vi "LC-MISDK_UserCalibration_MakeListData_XYZ.vi"(6 "Before_2":dbl, 7 "Before_3":dbl, 9 "before_1":dbl, 10 "タイムスタンプ":timestamp, 11 "Value":T1(ring)) -> (2 "リファレンス出力":refnum<k24>, 3 ".NET refnum出力":refnum<k24>)   [LabVIEW 2015]
uses:
  C:/Users/e09031/Documents/GMA/LC-160/Labview/Sample_LC-MISDK/LC-MISDK.dll
  LC-MISDK.dll
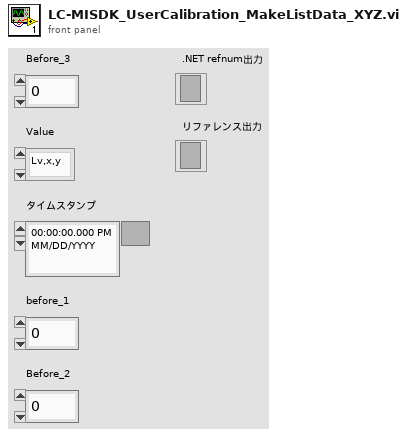
[diagram p1: front panel]
types:
  T1 = enum16{"Lv,x,y", "Lv,u',v'", "Lv,Tcp,duv", "X,Y,Z", "Lv,λd,Pe"}
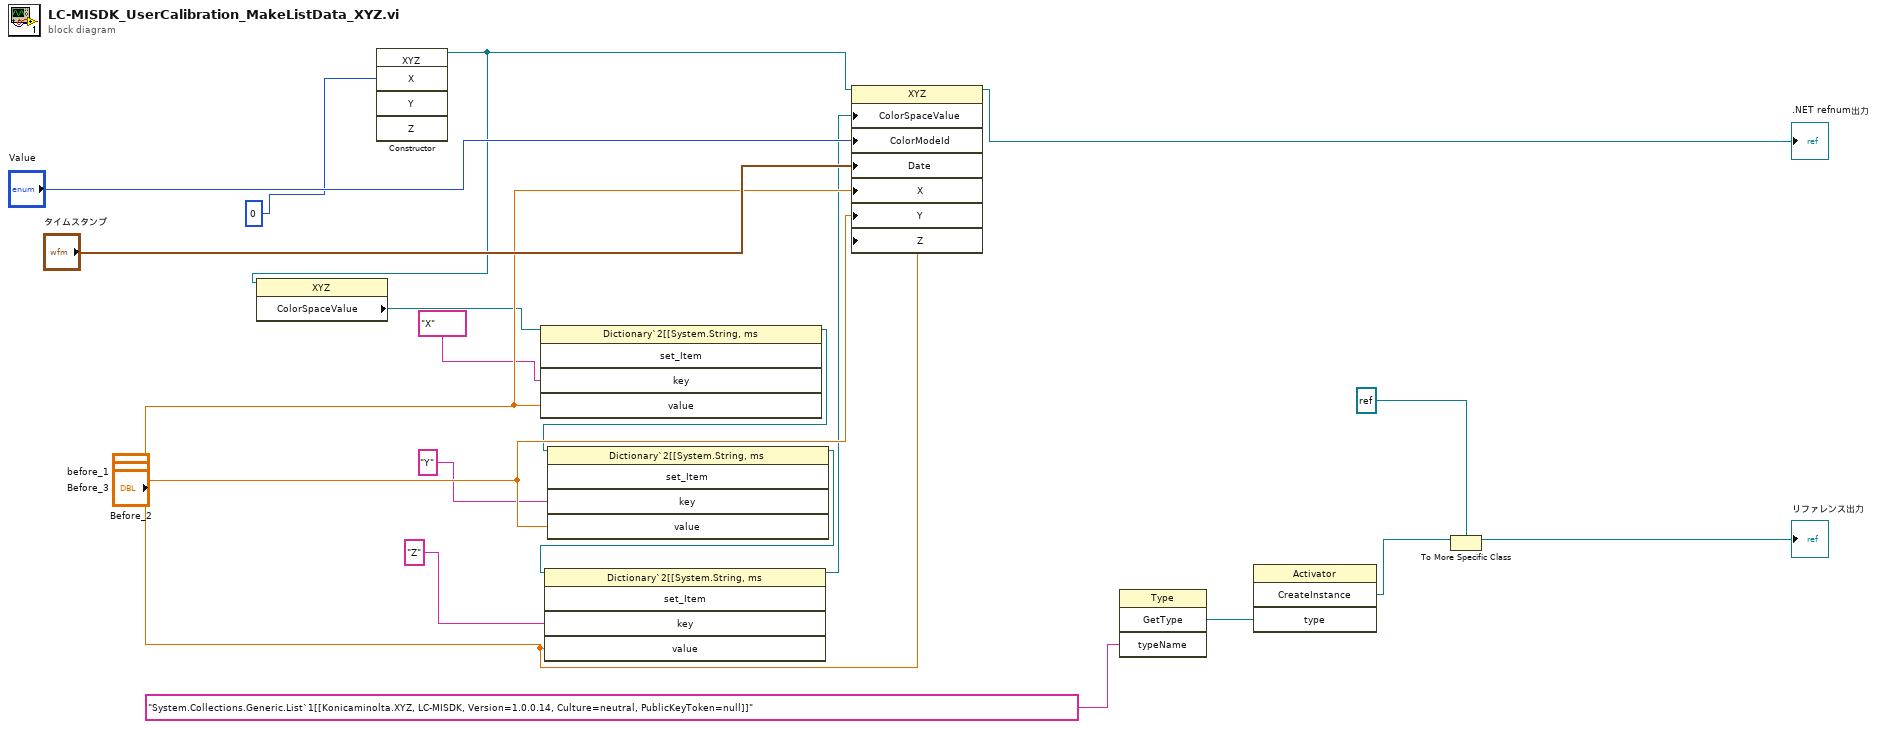
[diagram p0: block diagram]
diagram:
  n1 = constructor class="XYZ"("X"=0) -> (reference out=w8:refnum<k24>)  [unwired: 5 in, 5 out]
  n2 = property class="XYZ"(reference=w8) -> ("ColorSpaceValue"=w10:refnum<k24>)  [unwired: 1 in, 2 out]
  n3 = invoke on="インボークノード" class="Dictionary`2[[System.String, ms" method="set_Item"(reference=w10, "key"="X", "value"="before_1") -> (reference out=w4:refnum<k24>)  [unwired: 2 in, 4 out]
  n4 = invoke class="Dictionary`2[[System.String, ms" method="set_Item"(reference=w4, "key"="Y", "value"="Before_2") -> (reference out=w5:refnum<k24>)  [unwired: 2 in, 4 out]
  n5 = invoke class="Dictionary`2[[System.String, ms" method="set_Item"(reference=w5, "key"="Z", "value"="Before_3") -> (reference out=w7:refnum<k24>)  [unwired: 2 in, 4 out]
  n6 = property class="XYZ"(reference=w8, "ColorSpaceValue"=w7, "ColorModeId"="Value", "Date"="タイムスタンプ", "X"="before_1", "Y"="Before_2", "Z"="Before_3") -> (reference out=→".NET refnum出力":refnum<k24>)  [unwired: 1 in, 1 out]
  n7 = invoke on="インボークノード" class="Type" method="GetType"("typeName"="System.Collections.Generic.List`1[[Konicaminolta.XYZ, LC-MISDK, Version=1.0.0.14, Culture=neutral, PublicKeyToken=null]]") -> ("GetType"=w13:refnum<k24>)  [unwired: 3 in, 3 out]
  n8 = invoke on="インボークノード" class="Activator" method="CreateInstance"("type"=w13) -> ("CreateInstance"=w15:refnum<k24>)  [unwired: 3 in, 3 out]
  n9 = To More Specific Class(target class=refnum<k24> refnum ("リファレンス出力"), reference=w15) -> (specific class reference=→"リファレンス出力":refnum<k24>)  [unwired: 1 in, 1 out]
